vi "Edit_BSA_IP.vi"(3 "Show Panel":bool) -> (1 "Run LDA Diagnostic Out":bool)   [LabVIEW 2012]
uses:
  Controls/Beam_Power.ctl
  BSA_Type.ctl
  Globals/Meas_global.vi
  Globals/Constants_global.vi
  Globals/LDA_meas_global_1.vi
  Globals/LDA_meas_global_2.vi
panel:
  in  "BSA Type":T1
  in  "45 Degree Mirror":bool
  in  "Beam Alignment":u16(ring) items=["No Info", "Tunnel", "Model"]
  in  "Warn if Power below (mW)":T2
  out "Probe Options":string[](array[string])
  out "Green Fibre Separation":dbl[](array[numeric])
  out "Blue Fibre Separation":dbl[](array[numeric])
  in  "Cluster":cluster{"Focal Lengths":string[]}
  out "Focal Lengths Cluster":cluster{"Focal Lengths":string[]}[](array[cluster])
  out "Channel Values":string[][](array[string])
  out "Channel Names":string[](array[string])
  out "LDA_Probe_Information File":path
  in  "Focal Length 1":u16(ring) items=["160", "300"]
  in  "Focal Length 0":u16(ring) items=["160", "300"]
  in  "Non-coincident":bool
  in  "Run LDA Diagnostic":bool
  in  "Bandwidth 0":u16(ring)=11 items=["305.884", "152.942", "76.471", "38.235", "19.118", "9.559", "4.779", "2.390", "1.195", "0.597", "0.299", "0.149"]
  in  "Centre frequency 1":u16(ring)=20 items=["0.280", "0.261", "0.243", "0.224", "0.205", "0.187", "0.168", "0.149", "0.131", "0.112", "0.093", "0.075", "0.056", "0.037", "0.019", "0.000", "-0.019", "-0.037", "-0.056", "-0.075", "-0.093", "-0.112", "-0.131", "-0.149", "-0.168", "-0.187", "-0.205", "-0.224", "-0.243", "-0.261", "-0.280", "-0.299", "-0.317"]
  out "Record Length":dbl[](array[numeric])
  out "Final read?":bool
  in  "OK":bool
  out "C Array":dbl[](array[numeric])
  out "Bandwidth Array Hz":dbl[](array[numeric])
  in  "BSA IP Number":string
  in  "Bandwidth 1":u16(ring)=11 items=["305.726", "152.863", "76.431", "38.216", "19.108", "9.554", "4.777", "2.388", "1.194", "0.597", "0.299", "0.149"]
  in  "Centre frequency 0":u16(ring)=20 items=["-0.280", "-0.261", "-0.243", "-0.224", "-0.205", "-0.187", "-0.168", "-0.149", "-0.131", "-0.112", "-0.093", "-0.075", "-0.056", "-0.037", "-0.019", "-0.000", "0.019", "0.037", "0.056", "0.075", "0.093", "0.112", "0.131", "0.149", "0.168", "0.187", "0.205", "0.224", "0.243", "0.261", "0.280", "0.299", "0.317"]
  in  "Setup Array":T3(array[cluster]) {"Beams Colour" items=["Green Beams", "Blue Beams"]; "Fibre Colour" items=["Green Fibres", "Blue Fibres"]; "Probe Type" items=["27mm SN141", "27mm SN142"]; "Bandwidth Hz" format="%.3g"; "Min Record length" items=["16", "32", "64", "128", "256"]; "Optics Conversion Factor" format="%.3g"; "High voltage" min=0 max=2040 step=8; "Signal gain (dB)" min=0 max=30 step=1; "Max Record length" items=["16", "32", "64", "128", "256"]; "Min Velocity" format="%.2g"; "Max Velocity" format="%.2g"; "Wavelength (nm)" format="%.1f"}
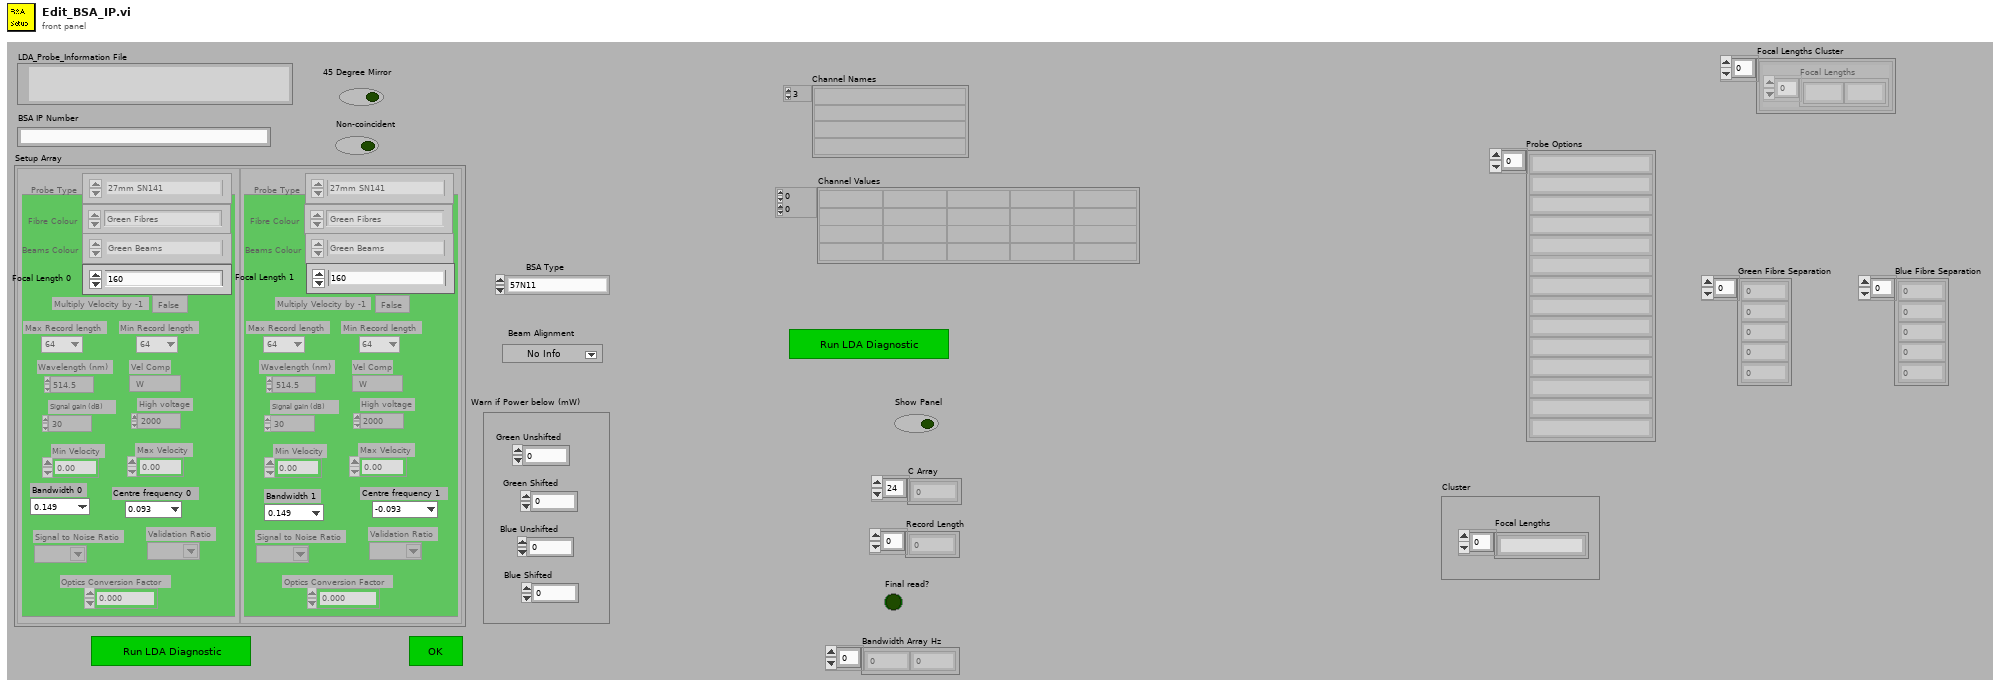
[diagram p1: front panel]
types:
  T1 = typedef "BSA_Type.ctl" = enum16{"57N11", "BSA F60"}
  T2 = typedef "Beam_Power.ctl" = cluster{"Green Unshifted":i32, "Green Shifted":i32, "Blue Unshifted":i32, "Blue Shifted":i32}
  T3 = cluster{"Wavelength (nm)":dbl, "Vel Comp":string, "Max Velocity":dbl, "Min Velocity":dbl, "COLOUR":u32, "Max Record length":u16, "Signal gain (dB)":i16, "High voltage":i16, "Optics Conversion Factor":dbl, "Min Record length":u16, "Bandwidth Hz":dbl, "Multiply Velocity by -1":bool, "Signal to Noise Ratio":string, "Validation Ratio":string, "Probe Type":u16, "Fibre Colour":u16, "Beams Colour":u16}[]
  T4 = typedef "LDA_Setup.ctl" = cluster{"dimensions":enum16{"1D", "2D"}, "Analogue Freq Multiplier":dbl}
  T5 = cluster{"Wavelength (nm)":dbl, "Vel Comp":string, "Max Velocity":dbl, "Min Velocity":dbl, "COLOUR":u32, "Max Record length":u16, "Signal gain (dB)":i16, "High voltage":i16, "Optics Conversion Factor":dbl, "Min Record length":u16, "Bandwidth Hz":dbl, "Multiply Velocity by -1":bool, "Signal to Noise Ratio":string, "Validation Ratio":string, "Probe Type":u16, "Fibre Colour":u16, "Beams Colour":u16}
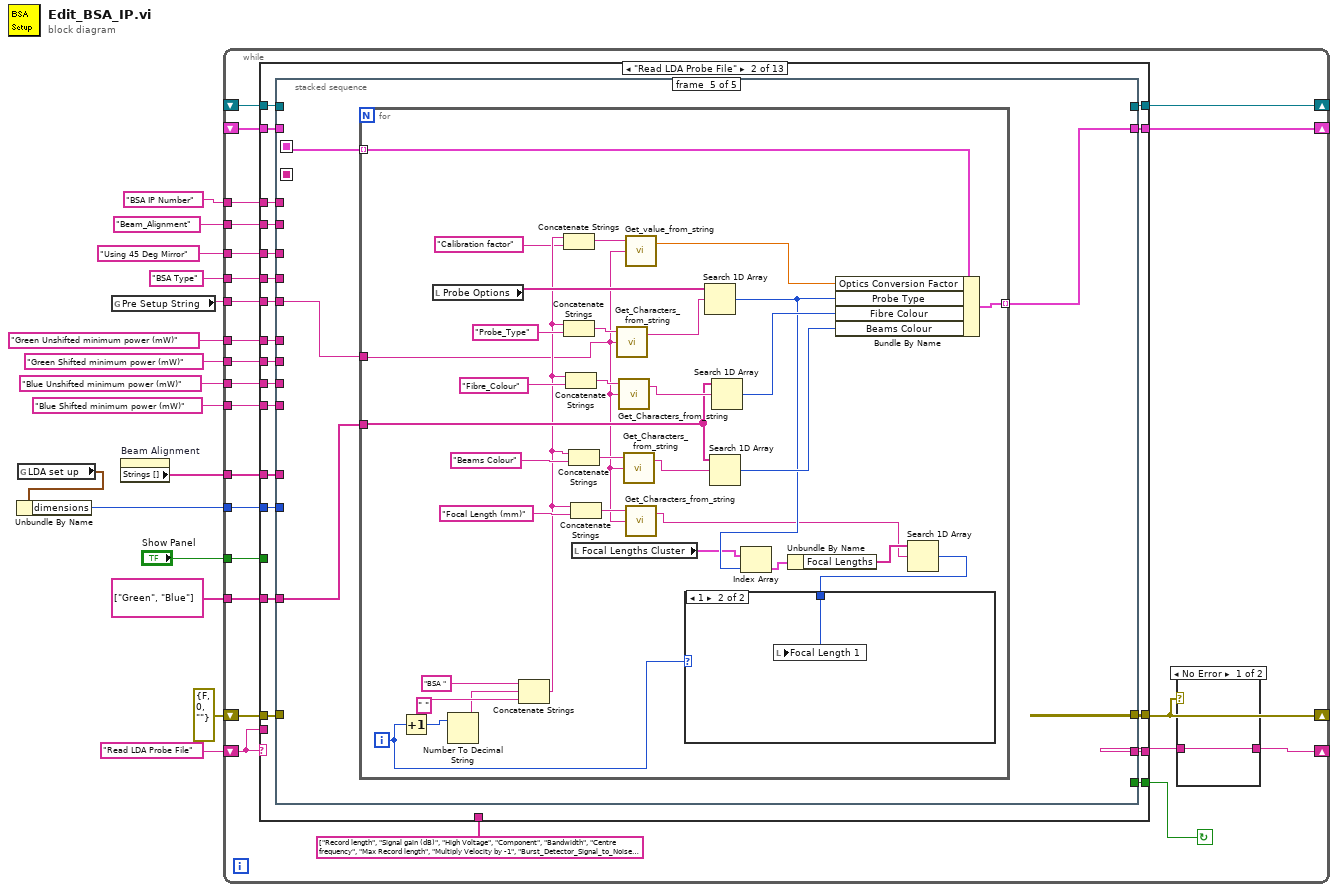
[diagram p0: block diagram]
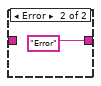
[diagram p2: hidden frame]
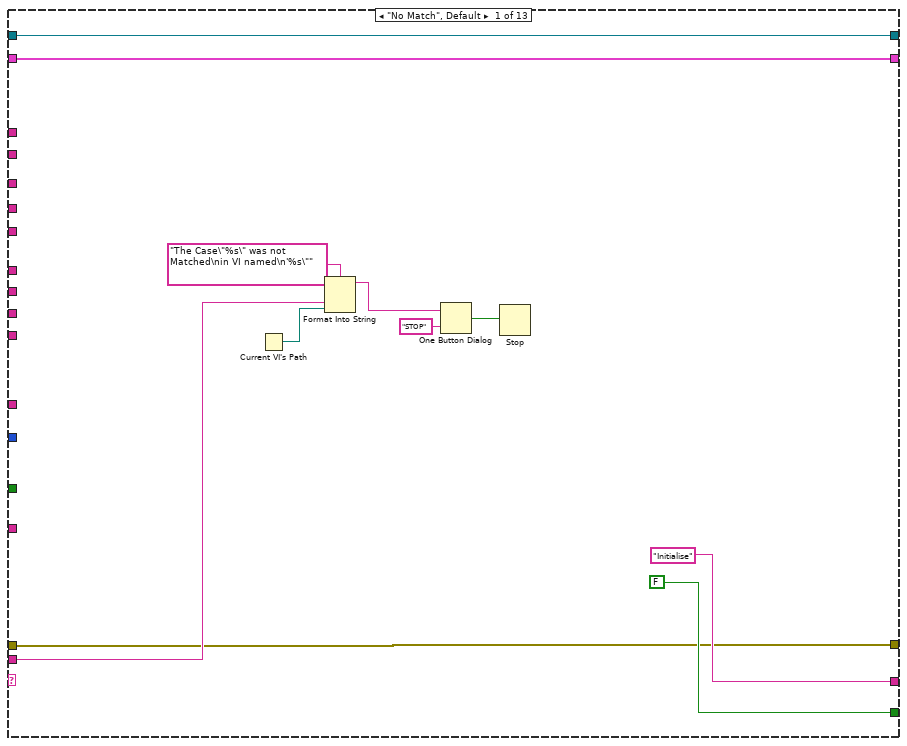
[diagram p3: hidden frame]
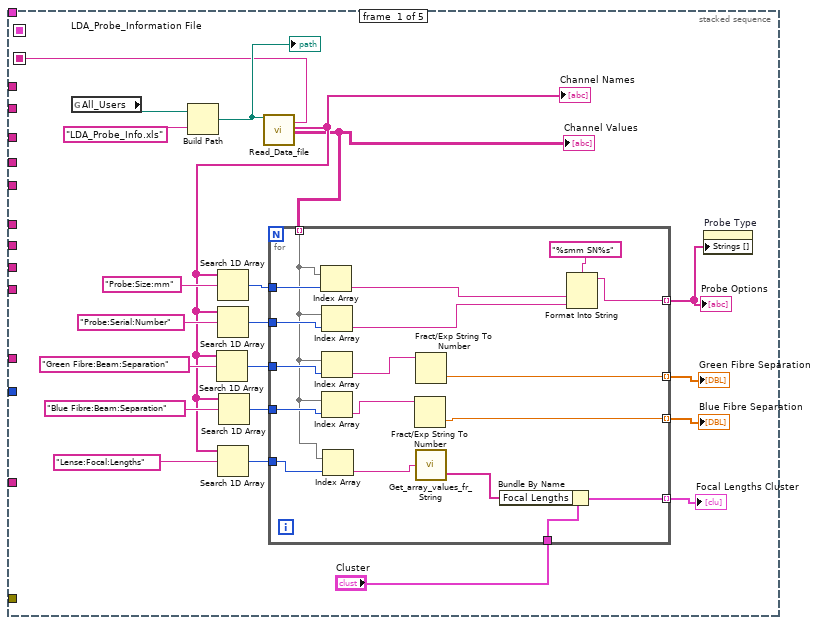
[diagram p4: hidden frame]
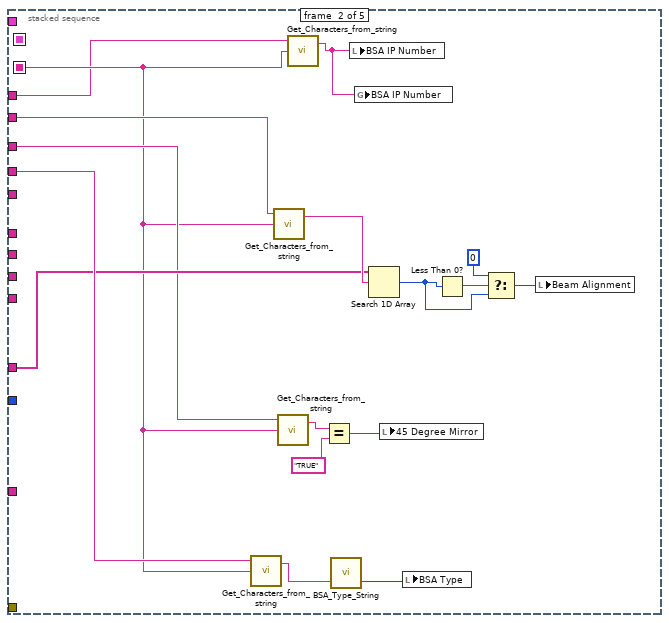
[diagram p5: hidden frame]
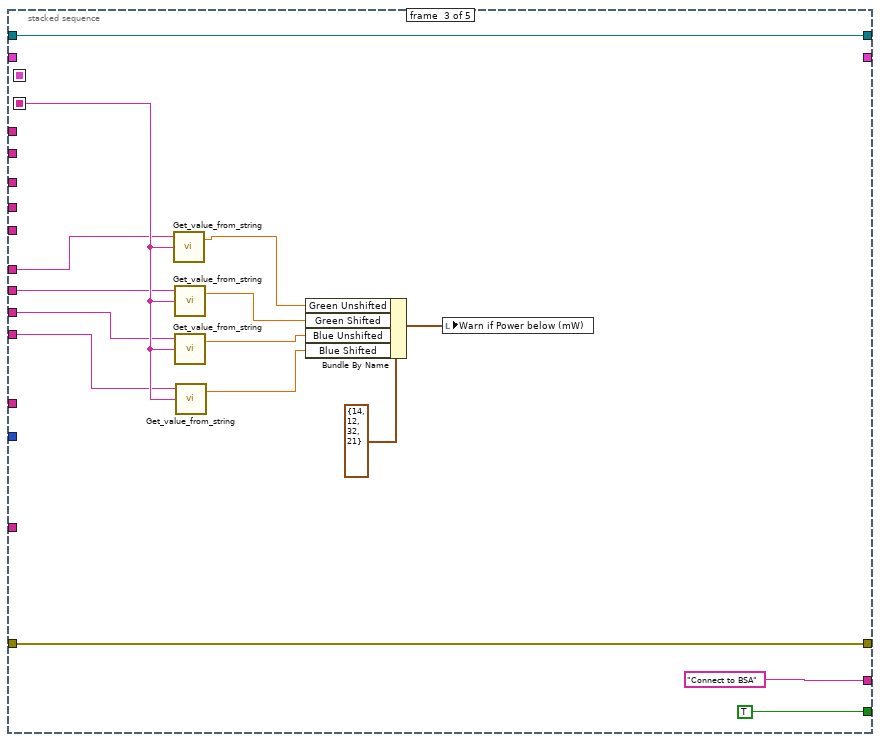
[diagram p6: hidden frame]
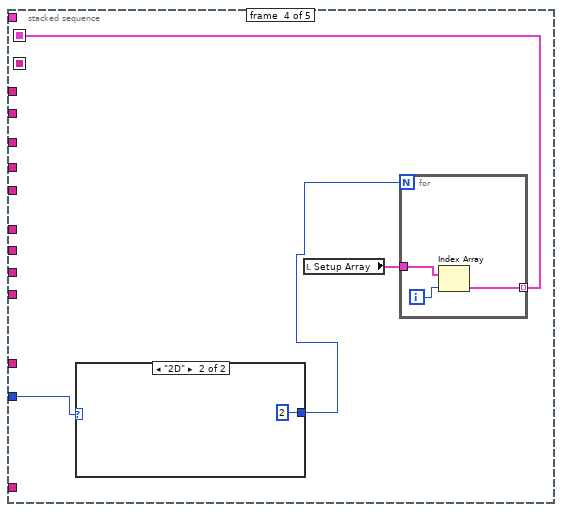
[diagram p7: hidden frame]
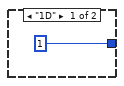
[diagram p8: hidden frame]
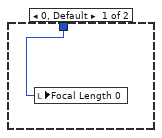
[diagram p9: hidden frame]
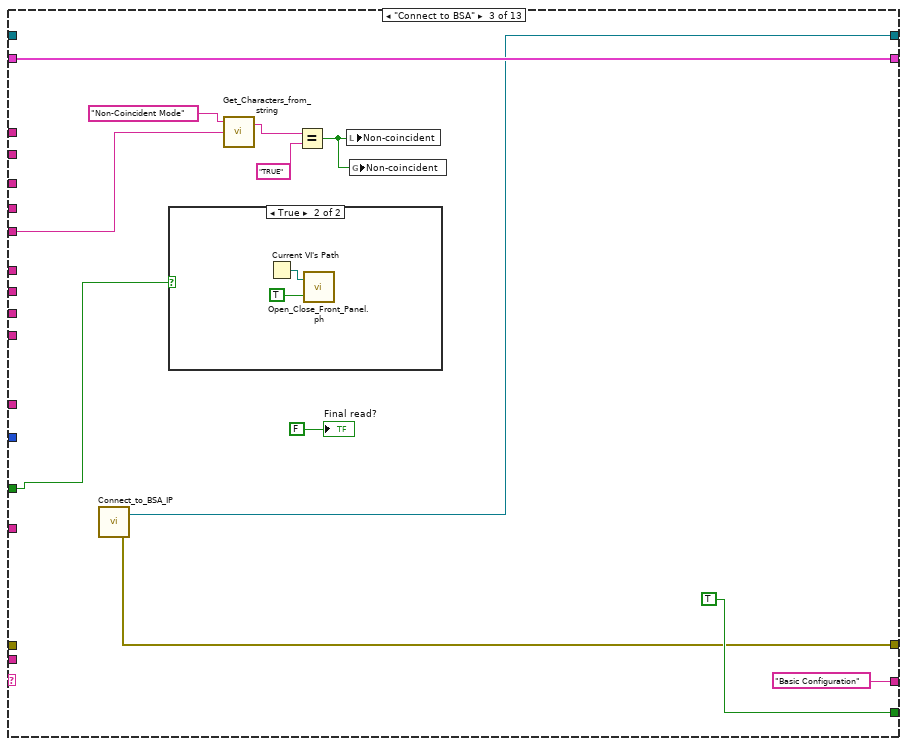
[diagram p10: hidden frame]
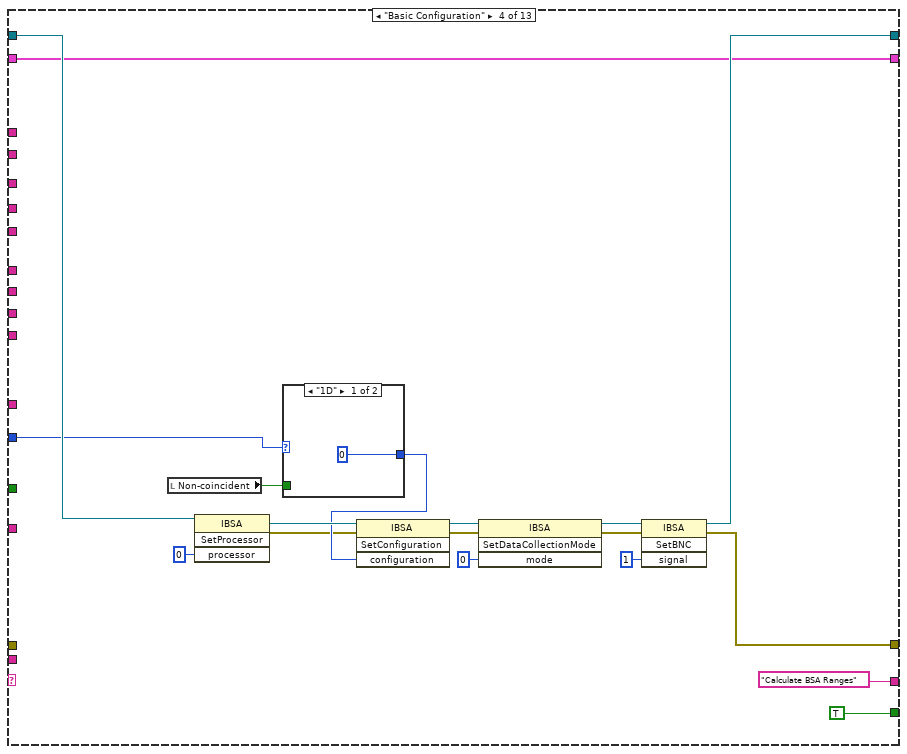
[diagram p12: hidden frame]
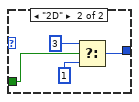
[diagram p13: hidden frame]
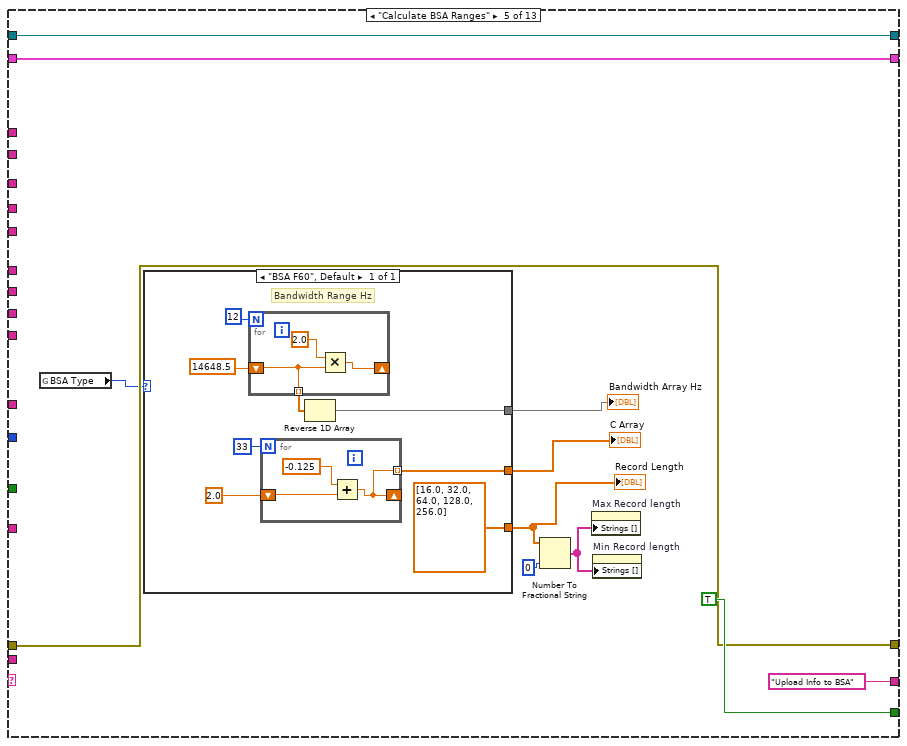
[diagram p14: hidden frame]
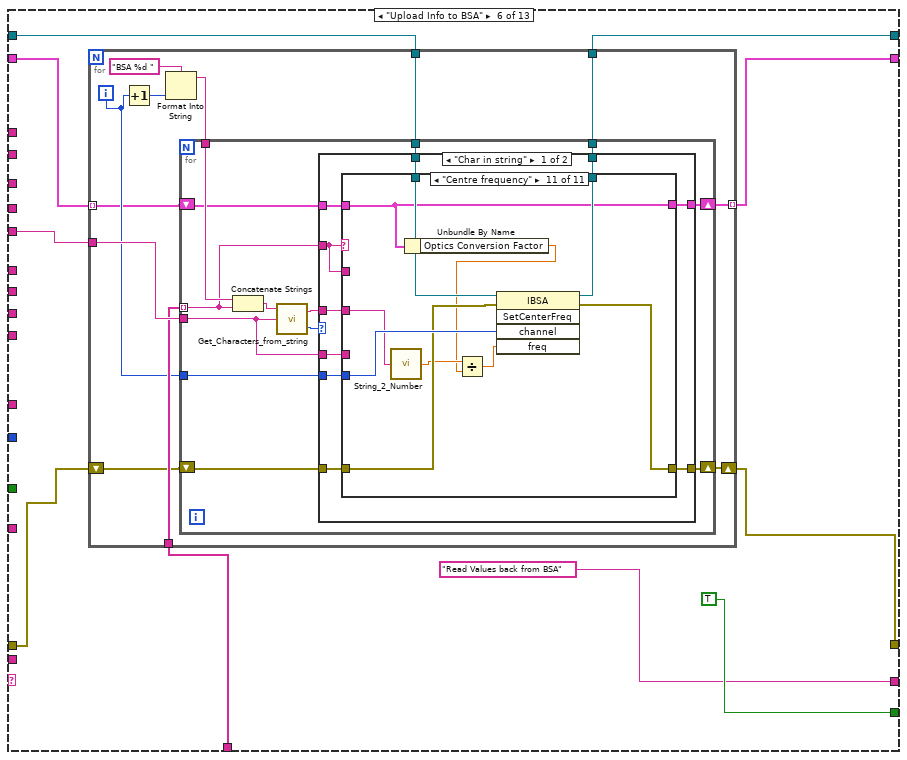
[diagram p15: hidden frame]
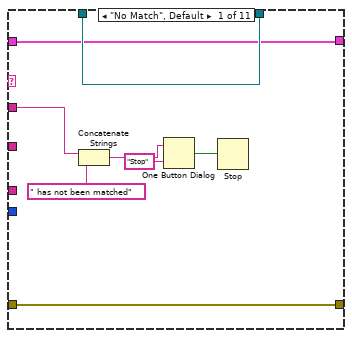
[diagram p16: hidden frame]
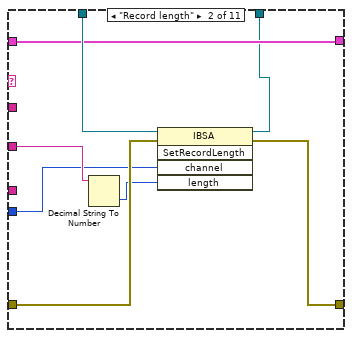
[diagram p17: hidden frame]
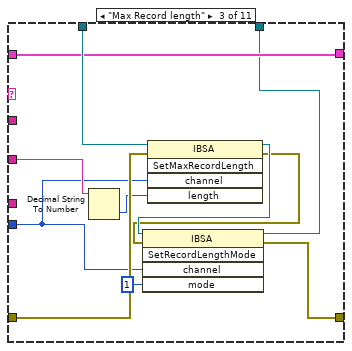
[diagram p18: hidden frame]
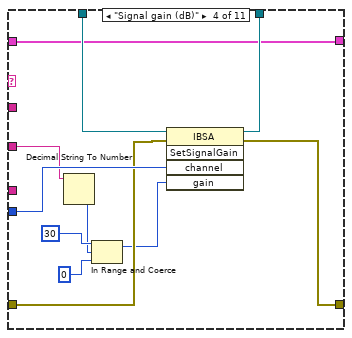
[diagram p19: hidden frame]
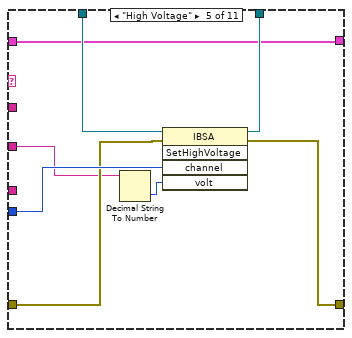
[diagram p20: hidden frame]
diagram:
  n1 = global read "Meas_global.vi" "LDA set up"() -> (w3:T4)
  n2 = Unbundle By Name(w3) -> ("dimensions"=w2:enum16{"1D", "2D"})
  n3 = global read "Meas_global.vi" "Pre Setup String"() -> (w15:string)
  n4 = property on="Beam Alignment" class="Ring (strict)"() -> ("Strings []"=w5:string[])  [unwired: 2 in, 2 out]
  n5 = while {
    shift-left: "Read LDA Probe File" -> [w39]
    shift-right: [w38] -> _
    shift-right: [w36] -> _
    shift-left: _ -> [w34]
    shift-right: [w28] -> _
    shift-left: errorcluster {"status"=FALSE, "code"=0, "source"=""} ("error out") -> [w35]
    tunnel: w15 -> [w33]
    shift-right: [w32] -> _
    shift-left: _ -> [w31]
    tunnel: "Show Panel" -> [w29]
    tunnel: "Green Unshifted minimum power (mW)" -> [w27]
    tunnel: "Green Shifted minimum power (mW)" -> [w26]
    tunnel: "Blue Unshifted minimum power (mW)" -> [w25]
    tunnel: "Blue Shifted minimum power (mW)" -> [w24]
    tunnel: "Using 45 Deg Mirror" -> [w23]
    tunnel: "BSA Type" -> [w22]
    tunnel: "Beam_Alignment" -> [w21]
    tunnel: "BSA IP Number" -> [w20]
    tunnel: w5 -> [w19]
    tunnel: string[] ["Green", "Blue"] -> [w18]
    tunnel: w2 -> [w17]
    stop <- w40 continue-if-true
    n6 = case shown="\"Read LDA Probe File\"" w39 {
      tunnel: [FALSE w72 TRUE TRUE TRUE TRUE TRUE TRUE TRUE ("Show Panel") TRUE FALSE TRUE ("Show Panel") w902] -> w40
      tunnel: ["Initialise" w73 "Basic Configuration" "Calculate BSA Ranges" "Upload Info to BSA" "Read Values back from BSA" w401 w539 w664 "Read Values back from BSA" "Second Case" "Write LDA Probe File" w899] -> w37
      tunnel: w39 -> [w48 _ _ _ _ _ _ _ _ _ _ _ _]
      tunnel: [w44 w70 w200 w211 w237 w259 w408 w544 w666 w684 w797 w807 w900] -> w28
      tunnel: [w45 w68 w201 w213 w239 w261 w410 w549 w670 w686 w798 w809 w895] -> w36
      tunnel: w35 -> [w44 w71 _ _ w237 w260 w409 w544 w666 w685 w797 w807 w901]
      tunnel: w34 -> [w45 w69 _ w219 w239 w262 w411 w549 w670 w687 w798 w809 w896]
      tunnel: w33 -> [_ w56 w197 _ _ w263 w412 _ _ w688 _ _ _]
      tunnel: [w43 w67 w202 w207 w238 w257 w405 w545 w663 w682 w796 w808 w897] -> w32
      tunnel: w31 -> [w43 w66 w202 w207 w238 w258 w407 _ w663 w683 w796 w808 w898]
      tunnel: string[] ["Record length", "Signal gain (dB)", "High Voltage", "Component", "Bandwidth", "Centre frequency", "Max Record length", "Multiply Velocity by -1", "Burst_Detector_Signal_to_Noise_Ratio", "Level_Validation_Ratio"] -> [_ _ _ _ _ w256 w406 _ _ w681 _ _ _]
      tunnel: w29 -> [_ _ w198 _ _ _ _ w536 _ _ _ _ w885]
      tunnel: w27 -> [_ w65 _ _ _ _ _ _ _ _ _ _ w894]
      tunnel: w26 -> [_ w64 _ _ _ _ _ _ _ _ _ _ w893]
      tunnel: w25 -> [_ w63 _ _ _ _ _ _ _ _ _ _ w892]
      tunnel: w24 -> [_ w62 _ _ _ _ _ _ _ _ _ _ w891]
      tunnel: w23 -> [_ w58 _ _ _ _ _ _ _ _ _ _ w890]
      tunnel: w22 -> [_ w61 _ _ _ _ _ _ _ _ _ _ w889]
      tunnel: w21 -> [_ w60 _ _ _ _ _ _ _ _ _ _ w888]
      tunnel: w20 -> [_ w57 _ _ _ _ _ _ _ _ _ _ w887]
      tunnel: w19 -> [_ w59 _ _ _ _ _ _ _ _ _ _ w886]
      tunnel: w18 -> [_ w55 _ _ _ _ _ _ _ _ _ w802 _]
      tunnel: w17 -> [_ w54 _ w208 _ _ _ _ _ _ _ _ _]
      frame "No Match", Default {
        n7 = Current VI's Path() -> (path=w47:path)
        n8 = Format Into String(format string="The Case\"%s\" was not Matched\nin VI named\n'%s\"" ("Format String"), w48, w47) -> (resulting string=w51:string)  [unwired: 2 in, 1 out]
        n9 = One Button Dialog(message=w51, button name ("OK")="STOP") -> (true=w49:bool)
        n10 = Stop(stop? (T)=w49) -> ()
      }
      frame "Read LDA Probe File" {
        n11 = stacked-sequence {
          seq-local: [w91 _ _ _ _] -> [_ w115 w134 _ _]
          seq-local: [_ _ _ w145 _] -> [_ _ _ _ w154]
          tunnel: [_ _ "Connect to BSA" _ _] -> w73
          tunnel: [_ _ TRUE ("Show Panel") _ _] -> w72
          tunnel: w71 -> [_ _ w142 _ _]
          tunnel: [_ _ w142 _ _] -> w70
          tunnel: w69 -> [_ _ w141 _ _]
          tunnel: [_ _ w141 _ _] -> w68
          tunnel: [_ _ _ _ w155] -> w67
          tunnel: w66 -> [_ _ _ _ _]
          tunnel: w65 -> [_ _ w133 _ _]
          tunnel: w64 -> [_ _ w132 _ _]
          tunnel: w63 -> [_ _ w131 _ _]
          tunnel: w62 -> [_ _ w130 _ _]
          tunnel: w61 -> [_ w127 _ _ _]
          tunnel: w60 -> [_ w122 _ _ _]
          tunnel: w59 -> [_ w121 _ _ _]
          tunnel: w58 -> [_ w117 _ _ _]
          tunnel: w57 -> [_ w114 _ _ _]
          tunnel: w56 -> [_ _ _ _ w157]
          tunnel: w55 -> [_ _ _ _ w156]
          tunnel: w54 -> [_ _ _ w147 _]
          frame #0 {
            n12 = global read "Constants_global.vi" "All_Users"() -> (w94:path)
            n13 = Build Path(base path=w94, name or relative path="LDA_Probe_Info.xls") -> (appended path=w92:path)
            "LDA_Probe_Information File" <- w92
            n14 = call "Read_Data_file.vi"("Results file"=w92) -> ("String Before"=w91:string, "Ch names Out"=w76:string[], "Channel Values Out"=w75:string[][])  [unwired: 9 in, 7 out]
            "Channel Names" <- w76
            "Channel Values" <- w75
            n15 = Search 1D Array(1D array=w76, element="Green Fibre:Beam:Separation") -> (index of element=w84:i32)  [unwired: 1 in]
            n16 = Search 1D Array(1D array=w76, element="Probe:Size:mm") -> (index of element=w79:i32)  [unwired: 1 in]
            n17 = Search 1D Array(1D array=w76, element="Probe:Serial:Number") -> (index of element=w80:i32)  [unwired: 1 in]
            n18 = Search 1D Array(1D array=w76, element="Lense:Focal:Lengths") -> (index of element=w88:i32)  [unwired: 1 in]
            n19 = Search 1D Array(1D array=w76, element="Blue Fibre:Beam:Separation") -> (index of element=w83:i32)  [unwired: 1 in]
            n20 = for {
              tunnel: w79 -> [w112]
              tunnel: w75 -> [w100] mode=indexing
              tunnel: w80 -> [w111]
              tunnel: [w107] -> w74 mode=indexing
              tunnel: w83 -> [w106]
              tunnel: w84 -> [w105]
              tunnel: [w102] -> w85 mode=indexing
              tunnel: [w101] -> w86 mode=indexing
              tunnel: w88 -> [w99]
              tunnel: "Cluster" -> [w97]
              tunnel: [w95] -> w90 mode=indexing
              n21 = Index Array(array=w100, index=w112) -> (element=w109:string)
              n22 = Index Array(array=w100, index=w111) -> (element=w108:string)
              n23 = Index Array(array=w100, index=w105) -> (element=w104:string)
              n24 = Index Array(array=w100, index=w106) -> (element=w103:string)
              n25 = Index Array(array=w100, index=w99) -> (element=w98:string)
              n26 = Fract/Exp String To Number(string=w103) -> (number=w101:dbl)  [unwired: 3 in, 1 out]
              n27 = Fract/Exp String To Number(string=w104) -> (number=w102:dbl)  [unwired: 3 in, 1 out]
              n28 = call "Get_array_values_fr_String.vi"("String Value"=w98) -> ("String array"=w96:string[])  [unwired: 1 out]
              n29 = Bundle By Name(cluster=w97, "Focal Lengths"=w96) -> (w95:cluster{"Focal Lengths":string[]})
              n30 = Format Into String(format string="%smm SN%s", w109, w108) -> (resulting string=w107:string)  [unwired: 2 in, 1 out]
            }
            "Probe Options" <- w74
            "Green Fibre Separation" <- w85
            "Blue Fibre Separation" <- w86
            "Focal Lengths Cluster" <- w90
            n31 = property on="Probe Type" class="Ring (strict)"("Strings []"=w74) -> ()  [unwired: 2 in, 2 out]
          }
          frame #1 {
            n32 = call "Get_Characters_from_string.vi"("Input string"=w115, "Variable name"=w127) -> ("Value"=w129:string)  [unwired: 1 in, 1 out]
            n33 = call "Get_Characters_from_string.vi"("Input string"=w115, "Variable name"=w122) -> ("Value"=w123:string)  [unwired: 1 in, 1 out]
            n34 = call "Get_Characters_from_string.vi"("Input string"=w115, "Variable name"=w117) -> ("Value"=w118:string)  [unwired: 1 in, 1 out]
            n35 = call "Get_Characters_from_string.vi"("Input string"=w115, "Variable name"=w114) -> ("Value"=w113:string)  [unwired: 1 in, 1 out]
            n36 = Equal?(x=w118, y="TRUE") -> (x = y?=w116:bool)
            n37 = call "BSA_Type_String.vi"("BSA String in"=w129) -> ("BSA Type Out"=w128:T1)  [unwired: 1 in, 1 out]
            n38 = local write "BSA IP Number"(w113) -> ()
            n39 = global write "LDA_meas_global_1.vi" "BSA IP Number"(w113) -> ()
            n40 = Search 1D Array(1D array=w121, element=w123) -> (index of element=w126:i32)  [unwired: 1 out]
            n41 = local write "45 Degree Mirror"(w116) -> ()
            n42 = local write "BSA Type"(w128) -> ()
            n43 = Less Than 0?(x=w126) -> (x < 0?=w124:bool)
            n44 = Select(t=0, s=w124, f=w126) -> (s? t:f=w120:i32)
            n45 = local write "Beam Alignment"(w120) -> ()
          }
          frame #2 {
            n46 = call "Get_value_from_string.vi"("Input string"=w134, "Variable name"=w133) -> ("Value"=w140:dbl)  [unwired: 1 in, 1 out]
            n47 = call "Get_value_from_string.vi"("Input string"=w134, "Variable name"=w132) -> ("Value"=w137:dbl)  [unwired: 1 in, 1 out]
            n48 = call "Get_value_from_string.vi"("Input string"=w134, "Variable name"=w131) -> ("Value"=w138:dbl)  [unwired: 1 in, 1 out]
            n49 = call "Get_value_from_string.vi"("Input string"=w134, "Variable name"=w130) -> ("Value"=w139:dbl)  [unwired: 1 in, 1 out]
            n50 = Bundle By Name(cluster=T2 {"Green Unshifted"=14, "Green Shifted"=12, "Blue Unshifted"=32, "Blue Shifted"=21} ("Warn if Power below (mW)"), "Green Unshifted"=w140, "Green Shifted"=w137, "Blue Unshifted"=w138, "Blue Shifted"=w139) -> (w136:T2)
            n51 = local write "Warn if Power below (mW)"(w136) -> ()
          }
          frame #3 {
            n52 = case shown="\"2D\"" w147 {
              tunnel: [1 2] -> w146
              frame "1D" {
              }
              frame "2D" {
              }
            }
            n53 = local read "Setup Array"() -> (w148:T3)
            n54 = for {
              N: w146 -> [_]
              tunnel: w148 -> [w152]
              tunnel: [w151] -> w145 mode=indexing
              i -> [w153]
              n55 = Index Array(array=w152, index=w153) -> (element=w151:T5)
            }
          }
          frame #4 {
            n56 = for {
              tunnel: w154 -> [w186] mode=indexing
              tunnel: w157 -> [w160]
              tunnel: w156 -> [w175]
              tunnel: [w163] -> w155 mode=indexing
              i -> [w172]
              n57 = Increment(x=w172) -> (x+1=w189:i32)
              n58 = local read "Probe Options"() -> (w183:string[])
              n59 = Number To Decimal String(number=w189) -> (decimal integer string=w187:string)  [unwired: 1 out]
              n60 = Concatenate Strings("BSA ", w187, " ") -> (w162:string)
              n61 = Concatenate Strings(w162, "Calibration factor") -> (w159:string)
              n62 = Concatenate Strings(w162, "Probe_Type" ("Pre Setup String")) -> (w184:string)
              n63 = Concatenate Strings(w162, "Fibre_Colour" ("string")) -> (w181:string)
              n64 = Concatenate Strings(w162, "Beams Colour") -> (w176:string)
              n65 = Concatenate Strings(w162, "Focal Length (mm)") -> (w168:string)
              n66 = local read "Focal Lengths Cluster"() -> (w169:cluster{"Focal Lengths":string[]}[])
              n67 = call "Get_Characters_from_string.vi"("Input string"=w160, "Variable name"=w184) -> ("Value"=w182:string)  [unwired: 1 in, 1 out]
              n68 = call "Get_Characters_from_string.vi"("Input string"=w160, "Variable name"=w181) -> ("Value"=w179:string)  [unwired: 1 in, 1 out]
              n69 = call "Get_Characters_from_string.vi"("Input string"=w160, "Variable name"=w176) -> ("Value"=w174:string)  [unwired: 1 in, 1 out]
              n70 = call "Get_value_from_string.vi"("Input string"=w160, "Variable name"=w159) -> ("Value"=w158:dbl)  [unwired: 1 in, 1 out]
              n71 = call "Get_Characters_from_string.vi"("Input string"=w160, "Variable name"=w168) -> ("Value"=w165:string)  [unwired: 1 in, 1 out]
              n72 = Search 1D Array(1D array=w183, element=w182) -> (index of element=w170:i32)  [unwired: 1 in]
              n73 = Search 1D Array(1D array=w175, element=w174) -> (index of element=w173:i32)  [unwired: 1 in]
              n74 = Search 1D Array(1D array=w175, element=w179) -> (index of element=w178:i32)  [unwired: 1 in]
              n75 = Index Array(array=w169, index=w170) -> (element=w171:cluster{"Focal Lengths":string[]})
              n76 = Unbundle By Name(w171) -> ("Focal Lengths"=w166:string[])
              n77 = Bundle By Name(cluster=w186, "Optics Conversion Factor"=w158, "Probe Type"=w170, "Fibre Colour"=w178, "Beams Colour"=w173) -> (w163:T5)
              n78 = Search 1D Array(1D array=w166, element=w165) -> (index of element=w164:i32)  [unwired: 1 in]
              n79 = case shown="1" w172 {
                tunnel: w164 -> [w191 w192]
                frame 0, Default {
                  n80 = local write "Focal Length 0"(w191) -> ()
                }
                frame 1 {
                  n81 = local write "Focal Length 1"(w192) -> ()
                }
              }
            }
          }
        }
      }
      frame "Connect to BSA" {
        n82 = call "Connect_to_BSA_IP.vi"() -> ("error out"=w200:errorcluster, "BSA"=w201:refnum<k7>)  [unwired: 2 out]
        n83 = case shown="True" w198 {
          frame False {
          }
          frame True {
            n84 = Current VI's Path() -> (path=w205:path)
            n85 = call "Open_Close_Front_Panel.ph.vi"("Front Panel Window:Open"=TRUE, "VI path"=w205) -> ()  [unwired: 2 out]
          }
        }
        n86 = call "Get_Characters_from_string.vi"("Input string"=w197, "Variable name"="Non-Coincident Mode" ("Pre Setup String")) -> ("Value"=w195:string)  [unwired: 1 in, 1 out]
        n87 = Equal?(x=w195, y="TRUE") -> (x = y?=w193:bool)
        n88 = local write "Non-coincident"(w193) -> ()
        n89 = global write "LDA_meas_global_1.vi" "Non-coincident"(w193) -> ()
        "Final read?" <- FALSE ("Boolean")
      }
      frame "Basic Configuration" {
        n90 = local read "Non-coincident"() -> (w215:bool)
        n91 = invoke class="IBSA" method="SetProcessor"(reference=w219, "processor"=0) -> (reference out=w222:refnum<k7>, error out=w220:errorcluster)  [unwired: 2 in, 2 out]
        n92 = case shown="\"1D\"" w208 {
          tunnel: [0 ("config") w229] -> w221
          tunnel: w215 -> [_ w228]
          frame "1D" {
          }
          frame "2D" {
            n93 = Select(t=3, s=w228, f=1 ("config")) -> (s? t:f=w229:i32)
          }
        }
        n94 = invoke class="IBSA" method="SetConfiguration"(reference=w222, error in=w220, "configuration"=w221) -> (reference out=w218:refnum<k7>, error out=w217:errorcluster)  [unwired: 1 in, 2 out]
        n95 = invoke class="IBSA" method="SetDataCollectionMode"(reference=w218, error in=w217, "mode"=0) -> (reference out=w214:refnum<k7>, error out=w212:errorcluster)  [unwired: 1 in, 2 out]
        n96 = invoke class="IBSA" method="SetBNC"(reference=w214, error in=w212, "signal"=1) -> (reference out=w213:refnum<k7>, error out=w211:errorcluster)  [unwired: 1 in, 2 out]
      }
      frame "Calculate BSA Ranges" {
        n97 = global read "LDA_meas_global_1.vi" "BSA Type"() -> (w231:T1)
        n98 = case shown="\"BSA F60\", Default" w231 {
          tunnel: [w243] -> w235
          tunnel: [w242] -> w234
          tunnel: [dbl[] [16.0, 32.0, 64.0, 128.0, 256.0] ("Max Record Length")] -> w232
          frame "BSA F60", Default {
            # "Bandwidth Range Hz"
            n99 = for {
              N: 12 -> [_]
              shift-right: [w254] -> _
              shift-left: 14648.5 -> [w252]
              tunnel: [w252] -> w246 mode=indexing
              n100 = Multiply(x=2.0, y=w252) -> (x*y=w254:dbl)
            }
            n101 = for {
              N: 33 -> [_]
              shift-right: [w249] -> _
              shift-left: 2.0 -> [w251]
              tunnel: [w249] -> w243 mode=indexing
              n102 = Add(x=-0.125, y=w251) -> (x+y=w249:dbl)
            }
            n103 = Reverse 1D Array(array=w246) -> (reversed array=w242:dbl[])
          }
        }
        "C Array" <- w235
        "Bandwidth Array Hz" <- w234
        "Record Length" <- w232
        n104 = Number To Fractional String(number=w232, precision (6)=i16 0) -> (F-format string=w230:string[])  [unwired: 2 out]
        n105 = property on="Max Record length" class="Ring (strict)"("Strings []"=w230) -> ()  [unwired: 2 in, 2 out]
        n106 = property on="Min Record length" class="Ring (strict)"("Strings []"=w230) -> ()  [unwired: 2 in, 2 out]
      }
      frame "Upload Info to BSA" {
        n107 = for {
          tunnel: w263 -> [w276]
          tunnel: w262 -> [w275]
          tunnel: [w274] -> w261
          shift-right: [w271] -> w259
          shift-left: w260 -> [w272]
          tunnel: w256 -> [w273]
          tunnel: w258 -> [w266] mode=indexing
          tunnel: [w265] -> w257 mode=indexing
          i -> [w270]
          n108 = Increment(x=w270) -> (x+1=w269:i32)
          n109 = Format Into String(format string="BSA %d ", w269) -> (resulting string=w267:string)  [unwired: 2 in, 1 out]
          n110 = for {
            tunnel: w267 -> [w289]
            tunnel: w270 -> [w288]
            tunnel: w276 -> [w281]
            tunnel: w275 -> [w287]
            tunnel: [w286] -> w274
            tunnel: w273 -> [w285] mode=indexing
            shift-right: [w283] -> w271
            shift-left: w272 -> [w284]
            shift-right: [w277] -> w265
            shift-left: w266 -> [w278]
            n111 = Concatenate Strings(w289, w285) -> (w282:string)
            n112 = call "Get_Characters_from_string.vi"("Input string"=w281, "Variable name"=w282) -> ("Status"=w280:enum16{"Char in string", "Char not in string"}, "Value"=w279:string)  [unwired: 1 in]
            n113 = case shown="\"Char in string\"" w280 {
              tunnel: w288 -> [w299 _]
              tunnel: w279 -> [w298 _]
              tunnel: w285 -> [w293 _]
              tunnel: w287 -> [w297 w400]
              tunnel: [w296 w400] -> w286
              tunnel: [w295 w399] -> w283
              tunnel: w284 -> [w294 w399]
              tunnel: w278 -> [w292 w398]
              tunnel: w281 -> [w291 _]
              tunnel: [w290 w398] -> w277
              frame "Char in string" {
                n114 = case shown="\"Centre frequency\"" w293 {
                  tunnel: w299 -> [_ w310 w320 w337 w345 w351 w360 w368 _ w387 w397]
                  tunnel: w298 -> [_ w313 w324 w332 w339 w353 w358 w366 w375 w382 w392]
                  tunnel: w297 -> [w307 w315 w326 w336 w344 w347 w362 w370 w371 w386 w396]
                  tunnel: [w307 w309 w316 w335 w343 w348 w355 w363 w371 w385 w395] -> w296
                  tunnel: [w306 w308 w317 w334 w342 w349 w356 w364 w372 w384 w394] -> w295
                  tunnel: w294 -> [w306 w314 w325 w333 w341 w346 w361 w369 w372 w383 w393]
                  tunnel: w293 -> [w305 _ _ _ _ _ _ _ _ _ _]
                  tunnel: w292 -> [w300 w312 w323 w331 w338 w354 w359 w367 w377 w380 w390]
                  tunnel: w291 -> [_ _ _ _ _ _ _ _ _ _ _]
                  tunnel: [w300 w312 w323 w331 w338 w352 w359 w367 w376 w380 w390] -> w290
                  frame "No Match", Default {
                    n115 = Concatenate Strings(w305, " has not been matched" ("string")) -> (w303:string)
                    n116 = One Button Dialog(message=w303, button name ("OK")="Stop") -> (true=w301:bool)
                    n117 = Stop(stop? (T)=w301) -> ()
                  }
                  frame "Record length" {
                    n118 = Decimal String To Number(string=w313) -> (number=w311:i32)  [unwired: 3 out]
                    n119 = invoke class="IBSA" method="SetRecordLength"(reference=w315, error in=w314, "channel"=w310, "length"=w311) -> (reference out=w309:refnum<k7>, error out=w308:errorcluster)  [unwired: 1 in, 3 out]
                  }
                  frame "Max Record length" {
                    n120 = Decimal String To Number(string=w324) -> (number=w322:i32)  [unwired: 3 out]
                    n121 = invoke class="IBSA" method="SetMaxRecordLength"(reference=w326, error in=w325, "channel"=w320, "length"=w322) -> (reference out=w319:refnum<k7>, error out=w318:errorcluster)  [unwired: 1 in, 3 out]
                    n122 = invoke class="IBSA" method="SetRecordLengthMode"(reference=w319, error in=w318, "channel"=w320, "mode"=1) -> (reference out=w316:refnum<k7>, error out=w317:errorcluster)  [unwired: 1 in, 3 out]
                  }
                  frame "Signal gain (dB)" {
                    n123 = Decimal String To Number(string=w332) -> (number=w327:i32)  [unwired: 3 out]
                    n124 = In Range and Coerce(upper limit=30, x=w327, lower limit=0) -> (coerced(x)=w328:i32)  [unwired: 1 out]
                    n125 = invoke class="IBSA" method="SetSignalGain"(reference=w336, error in=w333, "channel"=w337, "gain"=w328) -> (reference out=w335:refnum<k7>, error out=w334:errorcluster)  [unwired: 1 in, 3 out]
                  }
                  frame "High Voltage" {
                    n126 = Decimal String To Number(string=w339) -> (number=w340:i32)  [unwired: 3 out]
                    n127 = invoke class="IBSA" method="SetHighVoltage"(reference=w344, error in=w341, "channel"=w345, "volt"=w340) -> (reference out=w343:refnum<k7>, error out=w342:errorcluster)  [unwired: 1 in, 3 out]
                  }
                  frame "Component" {
                    n128 = invoke class="IBSA" method="SetAnodeCurrentLimit"(reference=w347, error in=w346, "channel"=w351, "limit"=1500) -> (reference out=w348:refnum<k7>, error out=w349:errorcluster)  [unwired: 1 in, 3 out]
                    n129 = Bundle By Name(cluster=w354, "Vel Comp"=w353) -> (w352:T5)
                  }
                  frame "Level_Validation_Ratio" {
                    n130 = Decimal String To Number(string=w358) -> (number=w357:i32)  [unwired: 3 out]
                    n131 = invoke class="IBSA" method="SetLevelValidationRatio"(reference=w362, error in=w361, "channel"=w360, "ratio"=w357) -> (reference out=w355:refnum<k7>, error out=w356:errorcluster)  [unwired: 1 in, 3 out]
                  }
                  frame "Burst_Detector_Signal_to_Noise_Ratio" {
                    n132 = Decimal String To Number(string=w366) -> (number=w365:i32)  [unwired: 3 out]
                    n133 = invoke class="IBSA" method="SetBurstDetectorSNR"(reference=w370, error in=w369, "channel"=w368, "snr"=w365) -> (reference out=w363:refnum<k7>, error out=w364:errorcluster)  [unwired: 1 in, 3 out]
                  }
                  frame "Multiply Velocity by -1" {
                    n134 = Equal?(x="TRUE", y=w375) -> (x = y?=w373:bool)
                    n135 = Bundle By Name(cluster=w377, "Multiply Velocity by -1"=w373) -> (w376:T5)
                  }
                  frame "Bandwidth" {
                    n136 = call "String_2_Number.vi"("Value"=w382) -> ("Numeric"=w381:dbl)
                    n137 = Unbundle By Name(w380) -> ("Optics Conversion Factor"=w379:dbl)
                    n138 = Divide(x=w381, y=w379) -> (x/y=w378:dbl)
                    n139 = invoke class="IBSA" method="SetBandwidth"(reference=w386, error in=w383, "channel"=w387, "bandwidth"=w378) -> (reference out=w385:refnum<k7>, error out=w384:errorcluster)  [unwired: 1 in, 3 out]
                  }
                  frame "Centre frequency" {
                    n140 = call "String_2_Number.vi"("Value"=w392) -> ("Numeric"=w391:dbl)
                    n141 = Unbundle By Name(w390) -> ("Optics Conversion Factor"=w389:dbl)
                    n142 = Divide(x=w391, y=w389) -> (x/y=w388:dbl)
                    n143 = invoke class="IBSA" method="SetCenterFreq"(reference=w396, error in=w393, "channel"=w397, "freq"=w388) -> (reference out=w395:refnum<k7>, error out=w394:errorcluster)  [unwired: 1 in, 3 out]
                  }
                }
              }
              frame "Char not in string" {
              }
            }
          }
        }
      }
      frame "Read Values back from BSA" {
        n144 = for {
          tunnel: w412 -> [w422]
          tunnel: w411 -> [w421]
          tunnel: [w420] -> w410
          shift-right: [w417] -> w408
          shift-left: w409 -> [w418]
          tunnel: w406 -> [w419]
          tunnel: w407 -> [w416] mode=indexing
          tunnel: [w415] -> w405 mode=indexing
          i -> [w414]
          n145 = for {
            tunnel: w414 -> [w431]
            tunnel: w422 -> [w425]
            tunnel: w421 -> [w430]
            tunnel: [w429] -> w420
            tunnel: w419 -> [w428] mode=indexing
            shift-right: [w426] -> w417
            shift-left: w418 -> [w427]
            shift-right: [w423] -> w415
            shift-left: w416 -> [w424]
            n146 = case shown="\"Centre frequency\"" w428 {
              tunnel: w431 -> [_ w451 w463 w471 w480 w489 w497 _ _ w511 w526]
              tunnel: w430 -> [w439 w450 w462 w470 w479 w488 w496 w499 w502 w515 w530]
              tunnel: [w439 w449 w461 w469 w478 w487 w495 w499 w502 w514 w529] -> w429
              tunnel: [w438 w448 w460 w468 w477 w486 w494 w500 w503 w513 w528] -> w426
              tunnel: w427 -> [w438 w447 w459 w467 w476 w485 w493 w500 w503 w512 w527]
              tunnel: w428 -> [w437 _ _ _ _ _ _ _ _ _ _]
              tunnel: w424 -> [w432 w446 w458 w465 w475 w484 w492 w498 w501 w506 w522]
              tunnel: w425 -> [_ _ _ _ _ _ _ _ _ _ _]
              tunnel: [w432 w445 w457 w464 w474 w483 w491 w498 w501 w504 w522] -> w423
              frame "No Match", Default {
                n147 = Concatenate Strings(w437, " has not been matched" ("string")) -> (w435:string)
                n148 = One Button Dialog(message=w435, button name ("OK")="Stop") -> (true=w433:bool)
                n149 = Stop(stop? (T)=w433) -> ()
              }
              frame "Record length" {
                n150 = local read "Record Length"() -> (w442:dbl[])
                n151 = invoke class="IBSA" method="GetRecordLength"(reference=w450, error in=w447, "channel"=w451) -> (reference out=w449:refnum<k7>, error out=w448:errorcluster, "GetRecordLength"=w441:i32)  [unwired: 1 in, 1 out]
                n152 = Subtract(x=w442, y=w441) -> (x-y=w444:dbl[])
                n153 = Absolute Value(x=w444) -> (abs(x)=w443:dbl[])
                n154 = Array Max & Min(array=w443) -> (min index (indices)=w440:i32)  [unwired: 3 out]
                n155 = Bundle By Name(cluster=w446, "Min Record length"=w440) -> (w445:T5)
              }
              frame "Max Record length" {
                n156 = local read "Record Length"() -> (w454:dbl[])
                n157 = invoke class="IBSA" method="GetMaxRecordLength"(reference=w462, error in=w459, "channel"=w463) -> (reference out=w461:refnum<k7>, error out=w460:errorcluster, "GetMaxRecordLength"=w453:i32)  [unwired: 1 in, 1 out]
                n158 = Subtract(x=w454, y=w453) -> (x-y=w456:dbl[])
                n159 = Absolute Value(x=w456) -> (abs(x)=w455:dbl[])
                n160 = Array Max & Min(array=w455) -> (min index (indices)=w452:i32)  [unwired: 3 out]
                n161 = Bundle By Name(cluster=w458, "Max Record length"=w452) -> (w457:T5)
              }
              frame "Signal gain (dB)" {
                n162 = invoke class="IBSA" method="GetSignalGain"(reference=w470, error in=w467, "channel"=w471) -> (reference out=w469:refnum<k7>, error out=w468:errorcluster, "GetSignalGain"=w466:i32)  [unwired: 1 in, 1 out]
                n163 = Bundle By Name(cluster=w465, "Signal gain (dB)"=w466) -> (w464:T5)
              }
              frame "Burst_Detector_Signal_to_Noise_Ratio" {
                n164 = invoke class="IBSA" method="GetBurstDetectorSNR"(reference=w479, error in=w476, "channel"=w480) -> (reference out=w478:refnum<k7>, error out=w477:errorcluster, "GetBurstDetectorSNR"=w472:i32)  [unwired: 1 in, 1 out]
                n165 = Number To Decimal String(number=w472) -> (decimal integer string=w473:string)  [unwired: 1 out]
                n166 = Bundle By Name(cluster=w475, "Signal to Noise Ratio"=w473) -> (w474:T5)
              }
              frame "Level_Validation_Ratio" {
                n167 = invoke class="IBSA" method="GetLevelValidationRatio"(reference=w488, error in=w485, "channel"=w489) -> (reference out=w487:refnum<k7>, error out=w486:errorcluster, "GetLevelValidationRatio"=w481:i32)  [unwired: 1 in, 1 out]
                n168 = Number To Decimal String(number=w481) -> (decimal integer string=w482:string)  [unwired: 1 out]
                n169 = Bundle By Name(cluster=w484, "Validation Ratio"=w482) -> (w483:T5)
              }
              frame "High Voltage" {
                n170 = invoke class="IBSA" method="GetHighVoltage"(reference=w496, error in=w493, "channel"=w497) -> (reference out=w495:refnum<k7>, error out=w494:errorcluster, "GetHighVoltage"=w490:i32)  [unwired: 1 in, 1 out]
                n171 = Bundle By Name(cluster=w492, "High voltage"=w490) -> (w491:T5)
              }
              frame "Component" {
              }
              frame "Multiply Velocity by -1" {
              }
              frame "Bandwidth" {
                n172 = local read "Bandwidth Array Hz"() -> (w508:dbl[])
                n173 = invoke class="IBSA" method="GetBandwidth"(reference=w515, error in=w512, "channel"=w511) -> (reference out=w514:refnum<k7>, error out=w513:errorcluster, "GetBandwidth"=w505:sgl)  [unwired: 1 in, 1 out]
                n174 = Bundle By Name(cluster=w506, "Bandwidth Hz"=w505) -> (w504:T5)
                n175 = Subtract(x=w508, y=w505) -> (x-y=w510:dbl[])
                n176 = Absolute Value(x=w510) -> (abs(x)=w509:dbl[])
                n177 = Array Max & Min(array=w509) -> (min index (indices)=w507:i32)  [unwired: 3 out]
                n178 = case shown="1" w511 {
                  tunnel: w507 -> [w516 w517]
                  frame 0, Default {
                    n179 = local write "Bandwidth 0"(w516) -> ()
                  }
                  frame 1 {
                    n180 = local write "Bandwidth 1"(w517) -> ()
                  }
                }
              }
              frame "Centre frequency" {
                n181 = local read "C Array"() -> (w521:dbl[])
                n182 = Unbundle By Name(w522) -> ("Bandwidth Hz"=w519:dbl)
                n183 = invoke class="IBSA" method="GetCenterFreq"(reference=w530, error in=w527, "channel"=w526) -> (reference out=w529:refnum<k7>, error out=w528:errorcluster, "GetCenterFreq"=w520:sgl)  [unwired: 1 in, 1 out]
                n184 = Divide(x=w520, y=w519) -> (x/y=w518:dbl)
                n185 = Subtract(x=w521, y=w518) -> (x-y=w525:dbl[])
                n186 = Absolute Value(x=w525) -> (abs(x)=w524:dbl[])
                n187 = Array Max & Min(array=w524) -> (min index (indices)=w523:i32)  [unwired: 3 out]
                n188 = case shown="1" w526 {
                  tunnel: w523 -> [w531 w532]
                  frame 0, Default {
                    n189 = local write "Centre frequency 0"(w531) -> ()
                  }
                  frame 1 {
                    n190 = local write "Centre frequency 1"(w532) -> ()
                  }
                }
              }
            }
          }
        }
        n191 = local read "Final read?"() -> (w404:bool)
        n192 = local write "Setup Array"(w405) -> ()
        n193 = Select(t="Update Globals", s=w404, f="Loop") -> (s? t:f=w401:string)
      }
      frame "Loop" {
        n194 = local read "Focal Lengths Cluster"() -> (w533:cluster{"Focal Lengths":string[]}[])
        n195 = local read "Bandwidth Array Hz"() -> (w548:dbl[])
        n196 = local read "C Array"() -> (w547:dbl[])
        n197 = Wait Until Next ms Multiple(millisecond multiple=u32 300) -> ()  [unwired: 1 out]
        n198 = for {
          tunnel: w548 -> [w556]
          tunnel: w547 -> [w553]
          tunnel: [w555] -> w545 mode=indexing
          tunnel: "Setup Array" -> [w552] mode=indexing
          tunnel: w533 -> [w551]
          i -> [w554]
          # "cf"
          # "BS"
          # "FL"
          # "WL"
          n199 = stacked-sequence {
            seq-local: [w558 _ _ _ _ _] -> [_ _ _ w587 _ w657]
            seq-local: [_ w570 _ _ _ _] -> [_ _ _ w595 _ w654]
            seq-local: [_ _ w579 _ _ _] -> [_ _ _ w596 _ w653]
            seq-local: [_ _ _ w592 _ _] -> [_ _ _ _ w600 w656]
            seq-local: [_ _ _ _ w599 _] -> [_ _ _ _ _ w658]
            seq-local: [w557 _ _ _ _ _] -> [_ _ _ _ _ w651]
            tunnel: w556 -> [_ _ _ w591 w626 _]
            tunnel: [_ _ _ _ _ w652] -> w555
            tunnel: w554 -> [_ w572 _ w593 w623 w655]
            tunnel: w553 -> [_ _ _ _ w611 _]
            tunnel: w552 -> [w560 w569 w583 _ w601 _]
            tunnel: w551 -> [_ w565 _ _ _ _]
            frame #0 {
              n200 = Unbundle By Name(w560) -> ("Beams Colour"=w559:u16)
              n201 = case shown="0, Default" w559 {
                tunnel: [514.5 ("Wavelength (nm)") 488.0 ("Wavelength (nm)")] -> w558
                tunnel: [u32 6618880 u32 3091199] -> w557
                frame 0, Default {
                }
                frame 1 {
                }
              }
            }
            frame #1 {
              n202 = Unbundle By Name(w569) -> ("Probe Type"=w568:u16)
              n203 = Index Array(array=w565, index=w568) -> (element=w567:cluster{"Focal Lengths":string[]})
              n204 = Unbundle By Name(w567) -> ("Focal Lengths"=w566:string[])
              n205 = case shown="1" w572 {
                tunnel: [w574 w578] -> w571
                tunnel: w566 -> [w573 w577]
                frame 0, Default {
                  n206 = property on="Focal Length 0" class="Ring (strict)"("Strings []"=w573) -> ()  [unwired: 2 in, 2 out]
                  n207 = Index Array(array=w573, index="Focal Length 0") -> (element=w574:string)
                }
                frame 1 {
                  n208 = property on="Focal Length 1" class="Ring (strict)"("Strings []"=w577) -> ()  [unwired: 2 in, 2 out]
                  n209 = Index Array(array=w577, index="Focal Length 1") -> (element=w578:string)
                }
              }
              n210 = Fract/Exp String To Number(string=w571) -> (number=w570:dbl)  [unwired: 3 in, 1 out]
            }
            frame #2 {
              n211 = Unbundle By Name(w583) -> ("Fibre Colour"=w582:u16, "Probe Type"=w580:u16)
              n212 = case shown="1" w582 {
                tunnel: [w584 w585] -> w581
                frame 0, Default {
                  n213 = local read "Green Fibre Separation"() -> (w584:dbl[])
                }
                frame 1 {
                  n214 = local read "Blue Fibre Separation"() -> (w585:dbl[])
                }
              }
              n215 = Index Array(array=w581, index=w580) -> (element=w579:dbl)
            }
            frame #3 {
              n216 = Divide(x=w587, y=1000000000.0) -> (x/y=w586:dbl)
              n217 = formula code="cf=lam/2/(sin(atan(bs/(2*fl))));"("bs"=w596, "fl"=w595, "lam"=w586) -> ("cf"=w592:dbl)
              n218 = Multiply(x=w592, y=w591) -> (x*y=w590:dbl[])
              n219 = Number To Fractional String(number=w590, precision (6)=i16 3) -> (F-format string=w589:string[])  [unwired: 2 out]
              n220 = case shown="1" w593 {
                tunnel: w589 -> [w597 w598]
                frame 0, Default {
                  n221 = property on="Bandwidth 0" class="Ring (strict)"("Strings []"=w597) -> ()  [unwired: 2 in, 2 out]
                }
                frame 1 {
                  n222 = property on="Bandwidth 1" class="Ring (strict)"("Strings []"=w598) -> ()  [unwired: 2 in, 2 out]
                }
              }
            }
            frame #4 {
              n223 = Unbundle By Name(w601) -> ("Max Record length"=w616:u16, "Min Record length"=w618:u16, "Multiply Velocity by -1"=w610:bool)
              n224 = case shown="0, Default" w623 {
                tunnel: ["Bandwidth 0" "Bandwidth 1"] -> w627
                tunnel: ["Centre frequency 0" "Centre frequency 1"] -> w625
                frame 0, Default {
                }
                frame 1 {
                }
              }
              n225 = Greater Or Equal?(x=w616, y=w618) -> (x >= y?=w617:bool)
              n226 = case shown="False" w617 {
                tunnel: w601 -> [w639 w640]
                tunnel: w616 -> [w638 _]
                tunnel: [w637 w640] -> w615
                frame False {
                  n227 = Bundle By Name(cluster=w639, "Min Record length"=w638) -> (w637:T5)
                }
                frame True {
                }
              }
              n228 = Index Array(array=w626, index=w627) -> (element=w622:dbl)
              n229 = Multiply(x=w600, y=w622) -> (x*y=w620:dbl)
              n230 = Multiply(x=w611, y=w620) -> (x*y=w607:dbl[])
              n231 = Index Array(array=w607, index=w625) -> (element=w612:dbl)
              n232 = Divide(x=w620, y=2.0) -> (x/y=w613:dbl)
              n233 = Negate(x=w613) -> (-x=w614:dbl)
              n234 = Add(x=w614, y=w612) -> (x+y=w608:dbl)
              n235 = Add(x=w613, y=w612) -> (x+y=w609:dbl)
              n236 = case shown="False" w610 {
                tunnel: [w628 w634] -> w602
                tunnel: w609 -> [w628 w636]
                tunnel: [w630 w633] -> w603
                tunnel: w608 -> [w630 w635]
                tunnel: w607 -> [w629 w632]
                tunnel: [w629 w631] -> w606
                frame False {
                }
                frame True {
                  n237 = Negate(x=w635) -> (-x=w633:dbl)
                  n238 = Negate(x=w636) -> (-x=w634:dbl)
                  n239 = Negate(x=w632) -> (-x=w631:dbl[])
                }
              }
              n240 = Max & Min(x=w603, y=w602) -> (max(x,y)=w604:dbl, min(x,y)=w605:dbl)
              n241 = Bundle By Name(cluster=w615, "Max Velocity"=w604, "Min Velocity"=w605) -> (w599:T5)
              n242 = Number To Fractional String(number=w606, precision (6)=i16 3) -> (F-format string=w619:string[])  [unwired: 2 out]
              n243 = case shown="0, Default" w623 {
                tunnel: w620 -> [w643 w646]
                tunnel: w612 -> [w642 w645]
                tunnel: w619 -> [w641 w644]
                frame 0, Default {
                  n244 = global write "LDA_meas_global_1.vi" "Centre Freq BSA1"(w642) -> ()
                  n245 = global write "LDA_meas_global_1.vi" "Bandwidth BSA1"(w643) -> ()
                  n246 = property on="Centre frequency 0" class="Ring (strict)"("Strings []"=w641) -> ()  [unwired: 2 in, 2 out]
                }
                frame 1 {
                  n247 = global write "LDA_meas_global_2.vi" "Centre Freq BSA2"(w645) -> ()
                  n248 = global write "LDA_meas_global_2.vi" "Bandwidth BSA2"(w646) -> ()
                  n249 = property on="Centre frequency 1" class="Ring (strict)"("Strings []"=w644) -> ()  [unwired: 2 in, 2 out]
                }
              }
            }
            frame #5 {
              n250 = case shown="1" w655 {
                tunnel: w654 -> [w660 w662]
                tunnel: w653 -> [w659 w661]
                frame 0, Default {
                  n251 = global write "LDA_meas_global_1.vi" "Focal Length (mm)"(w660) -> ()
                  n252 = global write "LDA_meas_global_1.vi" "Beam Separation (mm)"(w659) -> ()
                }
                frame 1 {
                  n253 = global write "LDA_meas_global_2.vi" "Beam Separation 2 (mm)"(w661) -> ()
                  n254 = global write "LDA_meas_global_2.vi" "Focal Length 2 (mm)"(w662) -> ()
                }
              }
              n255 = Bundle By Name(cluster=w658, "Wavelength (nm)"=w657, "Optics Conversion Factor"=w656, "COLOUR"=w651) -> (w652:T5)
            }
          }
        }
        n256 = Not Equal?(x=w545, y="Setup Array") -> (x != y?=w546:bool)
        n257 = case shown="True" w546 {
          tunnel: w545 -> [_ w550]
          frame False {
          }
          frame True {
            n258 = local write "Setup Array"(w550) -> ()
          }
        }
        n259 = Compound Arithmetic op=AND(invert "Run LDA Diagnostic", invert "OK", w536) -> (w540:bool)
        n260 = Select(t="Loop", s=w540, f="Check Vel Component") -> (s? t:f=w539:string)
        "Run LDA Diagnostic Out" <- "Run LDA Diagnostic"
      }
      frame "Check Vel Component" {
        n261 = for {
          tunnel: w663 -> [w679] mode=indexing
          shift-right: [w677] -> _
          shift-left: "" -> [w678]
          tunnel: [w674] -> w668 mode=indexing
          n262 = Unbundle By Name(w679) -> ("Vel Comp"=w677:string)
          n263 = Empty String/Path?(string/path=w677) -> (empty?=w676:bool)
          n264 = Not Equal?(x=w677, y=w678) -> (x != y?=w675:bool)
          n265 = Compound Arithmetic op=AND(invert w676, w675) -> (w674:bool)
        }
        n266 = And Array Elements(Boolean array=w668) -> (logical AND=w667:bool)
        n267 = case shown="False" w667 {
          tunnel: ["Loop" "Write Setup to BSA" ("f")] -> w664
          frame False {
            n268 = One Button Dialog(message="The \"Vel Comp\" should not be blank or the same") -> ()  [unwired: 1 in, 1 out]
          }
          frame True {
          }
        }
      }
      frame "Write Setup to BSA" {
        n269 = for {
          tunnel: w688 -> [w699]
          tunnel: w687 -> [w698]
          tunnel: [w697] -> w686
          shift-right: [w694] -> w684
          shift-left: w685 -> [w695]
          tunnel: w681 -> [w696]
          tunnel: w683 -> [w692] mode=indexing
          tunnel: [w691] -> w682 mode=indexing
          i -> [w693]
          n270 = for {
            tunnel: w693 -> [w708]
            tunnel: w699 -> [w702]
            tunnel: w698 -> [w707]
            tunnel: [w706] -> w697
            tunnel: w696 -> [w705] mode=indexing
            shift-right: [w703] -> w694
            shift-left: w695 -> [w704]
            shift-right: [w700] -> w691
            shift-left: w692 -> [w701]
            n271 = case shown="\"Burst_Detector_Signal_to_Noise_Ratio\"" w705 {
              tunnel: w708 -> [_ w725 w734 w741 w748 w756 w764 _ _ w776 w788]
              tunnel: w707 -> [w716 w724 w733 w740 w747 w755 w763 w766 w769 w780 w793]
              tunnel: [w716 w723 w732 w739 w746 w754 w762 w766 w769 w779 w792] -> w706
              tunnel: [w715 w722 w731 w738 w745 w753 w761 w767 w770 w778 w791] -> w703
              tunnel: w704 -> [w715 w721 w730 w737 w744 w752 w760 w767 w770 w777 w790]
              tunnel: w705 -> [w714 _ _ _ _ _ _ _ _ _ _]
              tunnel: w701 -> [w709 w720 w729 w736 w743 w751 w759 w765 w768 w773 w789]
              tunnel: w702 -> [_ _ _ _ _ _ _ _ _ _ _]
              tunnel: [w709 w720 w729 w736 w743 w751 w759 w765 w768 w772 w789] -> w700
              frame "No Match", Default {
                n272 = Concatenate Strings(w714, " has not been matched" ("string")) -> (w712:string)
                n273 = One Button Dialog(message=w712, button name ("OK")="Stop") -> (true=w710:bool)
                n274 = Stop(stop? (T)=w710) -> ()
              }
              frame "Record length" {
                n275 = Unbundle By Name(w720) -> ("Min Record length"=w718:u16)
                n276 = local read "Record Length"() -> (w719:dbl[])
                n277 = Index Array(array=w719, index=w718) -> (element=w717:dbl)
                n278 = invoke class="IBSA" method="SetRecordLength"(reference=w724, error in=w721, "channel"=w725, "length"=w717) -> (reference out=w723:refnum<k7>, error out=w722:errorcluster)  [unwired: 1 in, 3 out]
              }
              frame "Max Record length" {
                n279 = Unbundle By Name(w729) -> ("Max Record length"=w727:u16)
                n280 = local read "Record Length"() -> (w728:dbl[])
                n281 = Index Array(array=w728, index=w727) -> (element=w726:dbl)
                n282 = invoke class="IBSA" method="SetMaxRecordLength"(reference=w733, error in=w730, "channel"=w734, "length"=w726) -> (reference out=w732:refnum<k7>, error out=w731:errorcluster)  [unwired: 1 in, 3 out]
              }
              frame "Signal gain (dB)" {
                n283 = Unbundle By Name(w736) -> ("Signal gain (dB)"=w735:i16)
                n284 = invoke class="IBSA" method="SetSignalGain"(reference=w740, error in=w737, "channel"=w741, "gain"=w735) -> (reference out=w739:refnum<k7>, error out=w738:errorcluster)  [unwired: 1 in, 3 out]
              }
              frame "High Voltage" {
                n285 = Unbundle By Name(w743) -> ("High voltage"=w742:i16)
                n286 = invoke class="IBSA" method="SetHighVoltage"(reference=w747, error in=w744, "channel"=w748, "volt"=w742) -> (reference out=w746:refnum<k7>, error out=w745:errorcluster)  [unwired: 1 in, 3 out]
              }
              frame "Level_Validation_Ratio" {
                n287 = Unbundle By Name(w751) -> ("Validation Ratio"=w750:string)
                n288 = Decimal String To Number(string=w750) -> (number=w749:i32)  [unwired: 3 out]
                n289 = invoke class="IBSA" method="SetLevelValidationRatio"(reference=w755, error in=w752, "channel"=w756, "ratio"=w749) -> (reference out=w754:refnum<k7>, error out=w753:errorcluster)  [unwired: 1 in, 3 out]
              }
              frame "Burst_Detector_Signal_to_Noise_Ratio" {
                n290 = Unbundle By Name(w759) -> ("Signal to Noise Ratio"=w758:string)
                n291 = Decimal String To Number(string=w758) -> (number=w757:i32)  [unwired: 3 out]
                n292 = invoke class="IBSA" method="SetBurstDetectorSNR"(reference=w763, error in=w760, "channel"=w764, "snr"=w757) -> (reference out=w762:refnum<k7>, error out=w761:errorcluster)  [unwired: 1 in, 3 out]
              }
              frame "Component" {
              }
              frame "Multiply Velocity by -1" {
              }
              frame "Bandwidth" {
                n293 = case shown="1" w776 {
                  tunnel: [w781 w782] -> w775
                  frame 0, Default {
                    n294 = local read "Bandwidth 0"() -> (w781:u16)
                  }
                  frame 1 {
                    n295 = local read "Bandwidth 1"() -> (w782:u16)
                  }
                }
                n296 = local read "Bandwidth Array Hz"() -> (w774:dbl[])
                n297 = Index Array(array=w774, index=w775) -> (element=w771:dbl)
                n298 = Bundle By Name(cluster=w773, "Bandwidth Hz"=w771) -> (w772:T5)
                n299 = invoke class="IBSA" method="SetBandwidth"(reference=w780, error in=w777, "channel"=w776, "bandwidth"=w771) -> (reference out=w779:refnum<k7>, error out=w778:errorcluster)  [unwired: 1 in, 3 out]
              }
              frame "Centre frequency" {
                n300 = case shown="1" w788 {
                  tunnel: [w794 w795] -> w787
                  frame 0, Default {
                    n301 = local read "Centre frequency 0"() -> (w794:u16)
                  }
                  frame 1 {
                    n302 = local read "Centre frequency 1"() -> (w795:u16)
                  }
                }
                n303 = Unbundle By Name(w789) -> ("Bandwidth Hz"=w784:dbl)
                n304 = local read "C Array"() -> (w786:dbl[])
                n305 = Index Array(array=w786, index=w787) -> (element=w785:dbl)
                n306 = Multiply(x=w784, y=w785) -> (x*y=w783:dbl)
                n307 = invoke class="IBSA" method="SetCenterFreq"(reference=w793, error in=w790, "channel"=w788, "freq"=w783) -> (reference out=w792:refnum<k7>, error out=w791:errorcluster)  [unwired: 1 in, 3 out]
              }
            }
          }
        }
        n308 = local write "Final read?"(TRUE ("Boolean")) -> ()
      }
      frame "Error" {
        n309 = call "EnFlo_Error_Handler.vi"("error in (no error)"=w797, "Dialog Box (T)"=TRUE) -> ()  [unwired: 1 in, 3 out]
      }
      frame "Update Globals" {
        n310 = local read "Probe Options"() -> (w804:string[])
        n311 = for {
          tunnel: w808 -> [w813] mode=indexing
          tunnel: w804 -> [w811]
          tunnel: w802 -> [w810]
          i -> [w812]
          n312 = stacked-sequence {
            seq-local: [w827 _] -> [_ w846]
            tunnel: w813 -> [w841 w860]
            tunnel: w812 -> [w836 w847]
            tunnel: w811 -> [w817 _]
            tunnel: w810 -> [w815 w844]
            frame #0 {
              n313 = Increment(x=w836) -> (x+1=w839:i32)
              n314 = Unbundle By Name(w841) -> ("Signal to Noise Ratio"=w833:string, "Validation Ratio"=w831:string, "Probe Type"=w824:u16, "Fibre Colour"=w816:u16)
              n315 = Number To Decimal String(number=w839) -> (decimal integer string=w837:string)  [unwired: 1 out]
              n316 = Index Array(array=w815, index=w816) -> (element=w814:string)
              n317 = Concatenate Strings("BSA ", w837, " ") -> (w820:string)
              n318 = Concatenate Strings(w820, "Burst_Detector_Signal_to_Noise_Ratio" ("Pre Setup String")) -> (w834:string)
              n319 = Concatenate Strings(w820, "Level_Validation_Ratio" ("Pre Setup String")) -> (w832:string)
              n320 = Concatenate Strings(w820, "Probe_Type" ("Pre Setup String")) -> (w825:string)
              n321 = Index Array(array=w817, index=w824) -> (element=w823:string)
              n322 = Concatenate Strings(w820, "Fibre_Colour" ("string")) -> (w821:string)
              n323 = call "Characters_to_string.vi"("Characters to write"=w833, "Label for characters"=w834) -> ("Output string"=w828:string)
              n324 = call "Characters_to_string.vi"("Characters to write"=w831, "Label for characters"=w832) -> ("Output string"=w829:string)
              n325 = call "Characters_to_string.vi"("Characters to write"=w814, "Label for characters"=w821) -> ("Output string"=w818:string)
              n326 = call "Characters_to_string.vi"("Characters to write"=w823, "Label for characters"=w825) -> ("Output string"=w822:string)
              n327 = Concatenate Strings(w828, w829, w822, w818) -> (w827:string)
            }
            frame #1 {
              n328 = Unbundle By Name(w860) -> ("Max Record length"=w852:u16, "Min Record length"=w854:u16, "Vel Comp"=w859:string, "Signal gain (dB)"=w858:i16, "High voltage"=w857:i16, "Max Velocity"=w856:dbl, "Min Velocity"=w855:dbl, "Optics Conversion Factor"=w849:dbl, "Multiply Velocity by -1"=w848:bool, "Wavelength (nm)"=w845:dbl, "Beams Colour"=w842:u16)
              n329 = local read "Record Length"() -> (w851:dbl[])
              n330 = Index Array(array=w844, index=w842) -> (element=w843:string)
              n331 = Index Array(array=w851, index=w852) -> (element=w850:dbl)
              n332 = Index Array(array=w851, index=w854) -> (element=w853:dbl)
              n333 = case shown="1" w847 {
                tunnel: w853 -> [w872 w884]
                tunnel: w859 -> [w871 w878]
                tunnel: w858 -> [w870 w879]
                tunnel: w857 -> [w869 w880]
                tunnel: w856 -> [w868 w881]
                tunnel: w855 -> [w867 w882]
                tunnel: w849 -> [w866 w883]
                tunnel: w850 -> [w865 w877]
                tunnel: w848 -> [w864 w876]
                tunnel: w846 -> [w863 w875]
                tunnel: w845 -> [w862 w874]
                tunnel: w843 -> [w861 w873]
                frame 0, Default {
                  n334 = global write "LDA_meas_global_1.vi" "Max Record length BSA1"(w865) -> ()
                  n335 = global write "LDA_meas_global_1.vi" "Vel Comp BSA1"(w871) -> ()
                  n336 = global write "LDA_meas_global_1.vi" "Optic Calib factor BSA1"(w866) -> ()
                  n337 = global write "LDA_meas_global_1.vi" "Record length BSA1"(w872) -> ()
                  n338 = global write "LDA_meas_global_1.vi" "Additional BSA1 Setup"(w863) -> ()
                  n339 = global write "LDA_meas_global_1.vi" "Multiply Velocity by -1"(w864) -> ()
                  n340 = global write "LDA_meas_global_1.vi" "Wavelength 1 (nm)"(w862) -> ()
                  n341 = global write "LDA_meas_global_1.vi" "Signal gain BSA1"(w870) -> ()
                  n342 = global write "LDA_meas_global_1.vi" "Beams Colour 1"(w861) -> ()
                  n343 = global write "LDA_meas_global_1.vi" "High Volt BSA1"(w869) -> ()
                  n344 = global write "LDA_meas_global_1.vi" "Max Vel BSA1"(w868) -> ()
                  n345 = global write "LDA_meas_global_1.vi" "Min Vel BSA1"(w867) -> ()
                }
                frame 1 {
                  n346 = global write "LDA_meas_global_2.vi" "Max Record length BSA2"(w877) -> ()
                  n347 = global write "LDA_meas_global_2.vi" "Optic Calib factor BSA2"(w883) -> ()
                  n348 = global write "LDA_meas_global_2.vi" "Additional BSA2 Setup"(w875) -> ()
                  n349 = global write "LDA_meas_global_2.vi" "Wavelength 2 (nm)"(w874) -> ()
                  n350 = global write "LDA_meas_global_2.vi" "Multiply Velocity by -1"(w876) -> ()
                  n351 = global write "LDA_meas_global_2.vi" "Record length BSA2"(w884) -> ()
                  n352 = global write "LDA_meas_global_2.vi" "Beams Colour 2"(w873) -> ()
                  n353 = global write "LDA_meas_global_2.vi" "Signal gain BSA2"(w879) -> ()
                  n354 = global write "LDA_meas_global_2.vi" "Vel Comp BSA2"(w878) -> ()
                  n355 = global write "LDA_meas_global_2.vi" "High Volt BSA2"(w880) -> ()
                  n356 = global write "LDA_meas_global_2.vi" "Max Vel BSA2"(w881) -> ()
                  n357 = global write "LDA_meas_global_2.vi" "Min Vel BSA2"(w882) -> ()
                }
              }
            }
          }
        }
        n358 = global write "LDA_meas_global_1.vi" "Non-coincident"("Non-coincident") -> ()
      }
      frame "Write LDA Probe File" {
        n359 = stacked-sequence {
          seq-local: [_ w927 _ _] -> [_ _ w939 _]
          seq-local: [w906 _ _ _] -> [_ _ w940 _]
          tunnel: [_ _ _ FALSE] -> w902
          tunnel: w901 -> [_ _ _ w957]
          tunnel: [_ _ _ w957] -> w900
          tunnel: [_ _ _ "End"] -> w899
          tunnel: w898 -> [_ _ _ w955]
          tunnel: [_ _ _ w955] -> w897
          tunnel: w896 -> [_ _ _ w954]
          tunnel: [_ _ _ w954] -> w895
          tunnel: w894 -> [_ w932 _ _]
          tunnel: w893 -> [_ w931 _ _]
          tunnel: w892 -> [_ w930 _ _]
          tunnel: w891 -> [_ w929 _ _]
          tunnel: w890 -> [w914 _ _ _]
          tunnel: w889 -> [w915 _ _ _]
          tunnel: w888 -> [w913 _ _ _]
          tunnel: w887 -> [w911 _ _ _]
          tunnel: w886 -> [w905 _ _ _]
          tunnel: w885 -> [_ _ w938 _]
          frame #0 {
            n360 = global write "LDA_meas_global_1.vi" "Using 45 Degree Mirror?"("45 Degree Mirror") -> ()
            n361 = Index Array(array=w905, index="Beam Alignment") -> (element=w912:string)
            n362 = call "BSA_Type_String.vi"("BSA Type"="BSA Type") -> ("BSA String Out"=w916:string)  [unwired: 1 in, 1 out]
            n363 = Select(t="TRUE", s="45 Degree Mirror", f="FALSE") -> (s? t:f=w921:string)
            n364 = call "Characters_to_string.vi"("Characters to write"="BSA IP Number", "Label for characters"=w911) -> ("Output string"=w910:string)
            n365 = call "Characters_to_string.vi"("Characters to write"=w916, "Label for characters"=w915) -> ("Output string"=w907:string)
            n366 = call "Characters_to_string.vi"("Characters to write"=w921, "Label for characters"=w914) -> ("Output string"=w908:string)
            n367 = call "Characters_to_string.vi"("Characters to write"=w912, "Label for characters"=w913) -> ("Output string"=w909:string)
            n368 = global write "LDA_meas_global_1.vi" "BSA IP Number"("BSA IP Number") -> ()
            n369 = Concatenate Strings(w910, w909, w908, w907) -> (w906:string)
          }
          frame #1 {
            w926 = "\r\n"
            w933 = "0" ("precision")
            n370 = Unbundle By Name("Warn if Power below (mW)") -> ("Green Unshifted"=w925:i32, "Green Shifted"=w924:i32, "Blue Unshifted"=w923:i32, "Blue Shifted"=w922:i32)
            n371 = call "Value_to_string.vi"("precision"=w933, "Value"=w925, "Label for value"=w932) -> ("Output string"=w934:string)
            n372 = call "Value_to_string.vi"("precision"=w933, "Value"=w924, "Label for value"=w931) -> ("Output string"=w935:string)
            n373 = call "Value_to_string.vi"("precision"=w933, "Value"=w923, "Label for value"=w930) -> ("Output string"=w936:string)
            n374 = call "Value_to_string.vi"("precision"=w933, "Value"=w922, "Label for value"=w929) -> ("Output string"=w937:string)
            n375 = Concatenate Strings(w926, w934, w935, w936, w937, w926) -> (w927:string)
            n376 = global write "LDA_meas_global_1.vi" "Min Green Unshifted Power mW"(w925) -> ()
            n377 = global write "LDA_meas_global_1.vi" "Min Green Shifted Power mW"(w924) -> ()
            n378 = global write "LDA_meas_global_1.vi" "Min Blue Unshifted Power mW"(w923) -> ()
            n379 = global write "LDA_meas_global_1.vi" "Min Blue Shifted Power mW"(w922) -> ()
          }
          frame #2 {
            n380 = case shown="True" w938 {
              tunnel: w940 -> [_ w944]
              tunnel: w939 -> [_ w943]
              frame False {
              }
              frame True {
                n381 = local read "LDA_Probe_Information File"() -> (w947:path)
                n382 = local read "Channel Values"() -> (w945:string[][])
                n383 = local read "Channel Names"() -> (w946:string[])
                n384 = Current VI's Path() -> (path=w941:path)
                n385 = Initialize Array("", 15) -> (w950:string[])
                n386 = call "Open_Close_Front_Panel.ph.vi"("Front Panel Window:Open"=FALSE, "VI path"=w941) -> ()  [unwired: 2 out]
                n387 = call "Asterisk_header.vi"("Channel names"=w950) -> ("Header string"=w949:string)
                n388 = Concatenate Strings(w944, w943, w949) -> (w948:string)
                n389 = call "Write_Ch_data_file.vi"("Header string"=w948, "exists?"=FALSE, "Channel Values"=w945, "Channel names"=w946, "Filename"=w947) -> ()  [unwired: 3 in, 4 out]
              }
            }
          }
          frame #3 {
          }
        }
      }
    }
    n390 = case shown="No Error" w28 {
      tunnel: [w41 "Error"] -> w38
      tunnel: w37 -> [w41 _]
      frame No Error {
      }
      frame Error {
      }
    }
  }
